vi "Read_No_of_rows_fr_start.vi"(3 "Start of read offset (chars.: 0)":i32, 4 "No Of Rows":i32, 5 "Filename":path) -> (0 "Values":string[][](array[string]), 2 "Channel names":string[](array[string]))   [LabVIEW 2010]
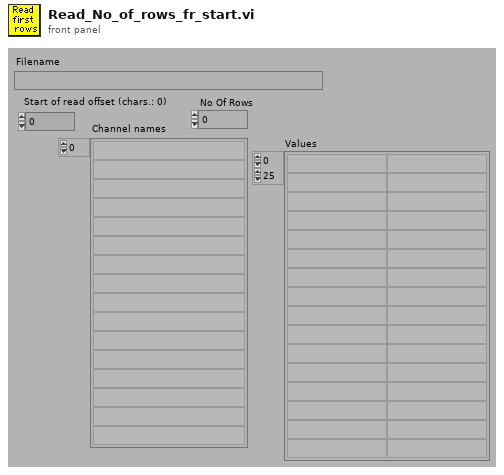
[diagram p1: front panel]
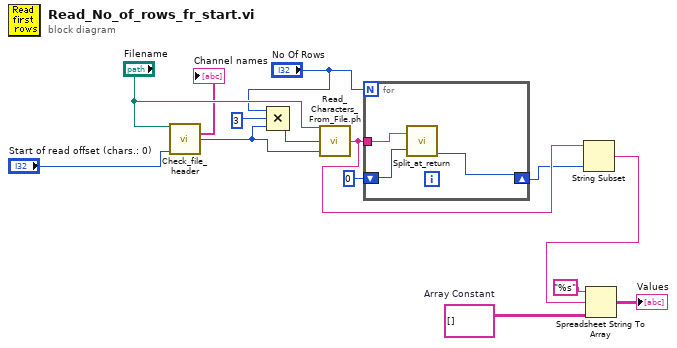
[diagram p0: block diagram]
diagram:
  w13 = string[][] []  # Array Constant
  n1 = call "Check_file_header.vi"("Filename"="Filename", "Start of read offset (chars.: 0)"="Start of read offset (chars.: 0)") -> ("Merged Channels"=→"Channel names":string[], "Start of data (bytes)"=w3:i32)  [unwired: 7 in, 5 out]
  n2 = Compound Arithmetic op=MULTIPLY("No Of Rows", 3 ("y"), w3) -> (w1:i32)
  n3 = call "Read_Characters_From_File.ph.vi"("file path (dialog if empty)"="Filename", "number of characters (all:-1)"=w1, "start of read offset (chars.: 0)"=w3) -> ("character string"=w8:string)  [unwired: 3 in, 3 out]
  n4 = for {
    N: "No Of Rows" -> [_]
    tunnel: w8 -> [w17]
    shift-right: [w15] -> w7
    shift-left: 0 ("offset past match") -> [w16]
    n5 = call "Split_at_return.vi"("String"=w17, "offset (0)"=w16) -> ("offset past match"=w15:i32)  [unwired: 3 out]
  }
  n6 = String Subset(string=w8, length (rest)=w7) -> (substring=w6:string)  [unwired: 1 in]
  n7 = Spreadsheet String To Array(format string="%s", spreadsheet string=w6, array type (2D Dbl)=w13) -> (array=→"Values":string[][])  [unwired: 1 in]
